vi "ExADCAsyncQ.vi"() -> ()   [LabVIEW 2010]
uses:
  Open-Close/CamHandle.vi
panel:
  in  "Intensifier":bool
  out "Pixel Time":i32
  out "Bit Depth":i32
  out "ReadOut port":i32
  out "ADC Offset":i32
  out "ADC Gain":i32
  out "ADC Speed":i32
  in  "Readout Port":i32=-1 min=-1 step=1
  in  "ADC Offset":i32=-1 min=-1 step=1
  in  "ADC Gain":i32=-1 min=-1 step=1
  in  "ADC speed":i32=-2 min=-3 step=1
  in  "Trigger Edge":u32(ring)=1 items=["N/A", "Positive (leading) edge", "Negative (falling) edge"]
  in  "Timing Mode":u32(ring)=1 items=["N/A", "Free Run/Timed", "Trigger First (PM only)", "Ext Sync/Strobed ", "Variable Exp (PM only)", "Flash Mode (PM only)"]
  in  "Temperature":dbl format="%.2f"
  in  "Exposure":dbl min=0.0 step=0.001 format="%.3f"
  out "error out":errorcluster
  in  "error in (no error)":errorcluster
  # "ExADCAsync:\nThis program shows how to use the  CameraADCset.vi and the CameraADCget.vi. This example allows all the ADC settings to be set or ignored."
  # "The following are read \nfrom camera after setting\nvalues to left.\n-1 value means it isn't \nsupported by camera."
  # "For Slowest ADC speed set this to -3\nFor Fastest ADC speed set this to -2\nTo use current ADC speed don't  hook up or use -1\notherwise put speed in as kHz"
  # "To use current gain don't hook up or set to -1"
  # "To use current gain don't hook up or set to -1"
  # "To use current gain don't hook up or set to -1"
  # "NOTICE\n\nTHIS VI USES A GLOBAL CAMERA HANDLE\n\nTHE VI EXOPENGLOBALCAM.VI MUST BE\nRUN AT THE START OF THE WORK SESSION.\nTHE CAMERA WILL REMAIN OPENED.\n\nTHE VI EXCLOSEGLOBALCAM.VI MUST\nBE RUN BEFORE LEAVING LABVIEW."
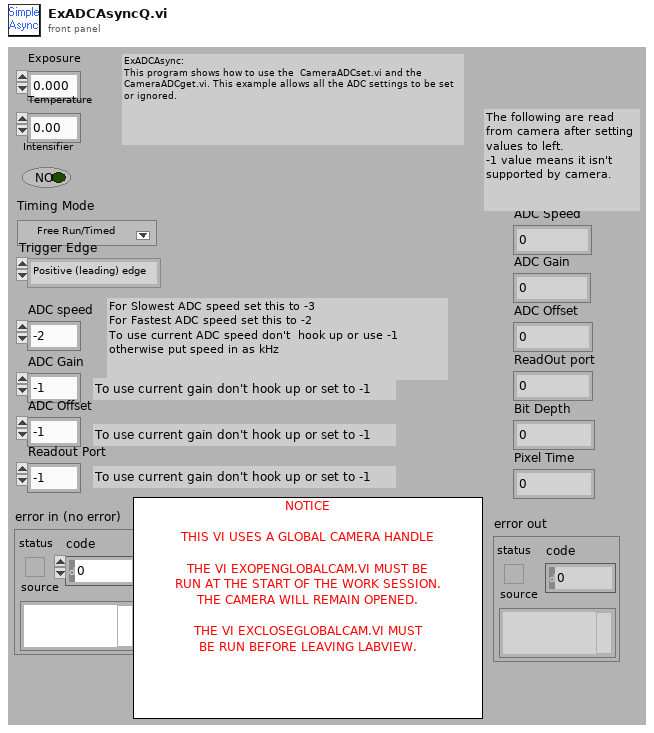
[diagram p1: front panel]
types:
  T1 = cluster{"Acquire mode \n3 is Async":i32, "Exposure":dbl, "Number of Images":i32, "Software Accums":i32}
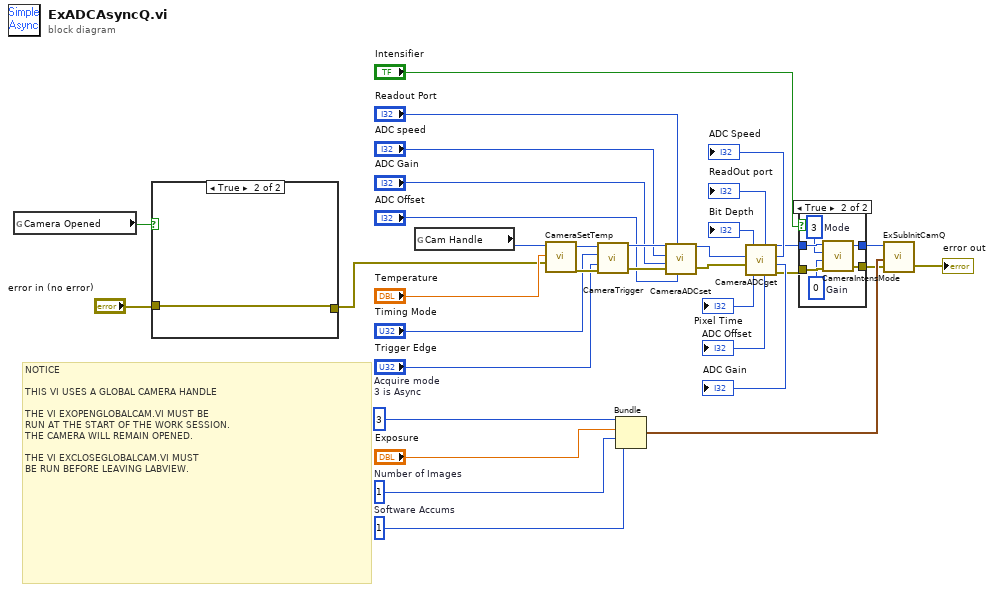
[diagram p0: block diagram]
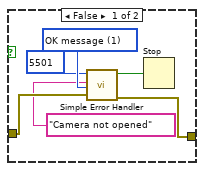
[diagram p2: hidden frame]
diagram:
  w33 = 1  # Number of Images
  w34 = 3  # Acquire mode  3 is Async
  w32 = 1  # Software Accums
  # "NOTICE\n\nTHIS VI USES A GLOBAL CAMERA HANDLE\n\nTHE VI EXOPENGLOBALCAM.VI MUST BE\nRUN AT THE START OF THE WORK SESSION.\nTHE CAMERA WILL REMAIN OPENED.\n\nTHE VI EXCLOSEGLOBALCAM.VI MUST\nBE RUN BEFORE LEAVING LABVIEW."
  n1 = global read "CamHandle.vi" "Camera Opened"() -> (w5:bool)
  n2 = case shown="True" w5 {
    tunnel: "error in (no error)" -> [w39 w41]
    tunnel: [w38 w41] -> w3
    frame False {
      w40 = u16 1 items=["no dialog", "OK message", "continue or stop message"] ("type of dialog (OK msg:1)")
      n3 = call <vilib>:"Simple Error Handler.vi"("error code (no error:0)"=5501, "error source (\" \")"="Camera not opened", "type of dialog (OK msg:1)"=w40, "error in (no error)"=w39) -> ("error?"=w36:bool, "error out"=w38:errorcluster)  [unwired: 1 in, 3 out]
      n4 = Stop(stop? (T)=w36) -> ()
    }
    frame True {
    }
  }
  n5 = global read "CamHandle.vi" "Cam Handle"() -> (w2:u32)
  n6 = call <userlib>:"CameraSetTemp.vi"("error in (no error)"=w3, "Temperature"="Temperature", "Camera Handle"=w2) -> ("error out"=w27:errorcluster, "Camera Handle"=w28:u32)
  n7 = call <userlib>:"CameraTrigger.vi"("error in"=w27, "Trigger Edge"="Trigger Edge", "Timing Mode"="Timing Mode", "Camera Handle"=w28) -> ("error out"=w15:errorcluster, "Camera Handle"=w16:u32)
  n8 = Bundle("Acquire mode \n3 is Async"=w34, "Exposure"="Exposure", "Number of Images"=w33, "Software Accums"=w32) -> (w30:T1)  [unwired: 1 in]
  n9 = call <userlib>:"CameraADCset.vi"("ADC offset"="ADC Offset", "Read Out port"="Readout Port", "error in (no error)"=w15, "ADC Gain"="ADC Gain", "ADC Speed"="ADC speed", "Camera Handle"=w16) -> ("error out"=w18:errorcluster, "Camera Handle"=w19:u32)
  n10 = call <userlib>:"CameraADCget.vi"("Camera handle"=w19, "error in (no error)"=w18) -> ("Bit Depth"=→"Bit Depth":i32, "Pixel Time"=→"Pixel Time":i32, "Readout Port"=→"ReadOut port":i32, "ADC Offset"=→"ADC Offset":i32, "Camera handle"=w7:u32, "ADC Speed"=→"ADC Speed":i32, "ADC Gain"=→"ADC Gain":i32, "error out"=w8:errorcluster)
  n11 = case shown="True" "Intensifier" {
    tunnel: w7 -> [w43 w49]
    tunnel: [w43 w48] -> w9
    tunnel: w8 -> [w42 w47]
    tunnel: [w42 w46] -> w10
    frame False {
    }
    frame True {
      w44 = u32 0  # Gain
      w45 = u32 3  # Mode
      n12 = call <userlib>:"CameraIntensMode.vi"("error in"=w47, "Intensifier Gain"=w44, "Mode"=w45, "Camera Handle"=w49) -> ("error out"=w46:errorcluster, "Camera Handle"=w48:u32)
    }
  }
  n13 = call "ExSubInitCamQ.vi"("error in (no error)"=w10, "Camera Information"=w30, "Camera Handle"=w9) -> ("error out"=→"error out":errorcluster)  [unwired: 1 out]
